vi "event_setup_start.vi"(7 "NewVal":bool, 8 "error in":errorcluster, 9 "reference cluster in":T1, 11 "Boolean in":refnum<vi>) -> (0 "error out":errorcluster)   [LabVIEW 2016]
uses:
  Type Definitions/reference_cluster.ctl
  Type Definitions/vars_settings.ctl
  Type Definitions/stim_type.ctl
  Type Definitions/backlight_type.ctl
  Type Definitions/vars_runtime.ctl
  Type Definitions/data.ctl
  Type Definitions/notifier_elements_GUI.ctl
  Type Definitions/notifier_elements_DAQ.ctl
  Type Definitions/notifier_elements_write.ctl
  Type Definitions/control_references.ctl
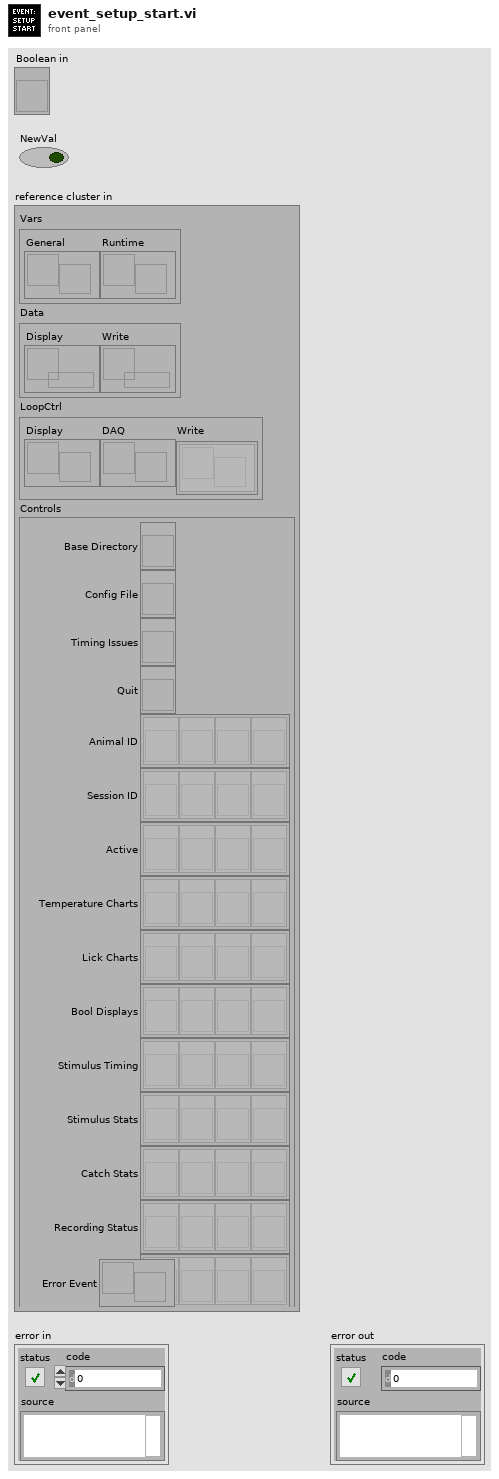
[diagram p1: front panel]
types:
  T1 = typedef "reference_cluster.ctl" = cluster{"Vars":cluster{"General":refnum<notifier>, "Runtime":refnum<notifier>}, "Data":cluster{"Display":refnum<queue>, "Write":refnum<queue>}, "LoopCtrl":cluster{"Display":refnum<notifier>, "DAQ":refnum<notifier>, "Write":refnum<notifier>[]}, "Controls":T2, "Error Event":refnum<user-event>}
  T2 = typedef "control_references.ctl" = cluster{"Base Directory":refnum<vi>, "Config File":refnum<vi>, "Timing Issues":refnum<vi>, "Quit":refnum<vi>, "Animal ID":refnum<vi>[], "Session ID":refnum<vi>[], "Active":refnum<vi>[], "Temperature Charts":refnum<vi>[], "Lick Charts":refnum<vi>[], "Bool Displays":refnum<vi>[], "Stimulus Timing":refnum<vi>[], "Stimulus Stats":refnum<vi>[], "Catch Stats":refnum<vi>[], "Recording Status":refnum<vi>[], "Pairing":refnum<vi>[]}
  T3 = enum8{"Enabled", "Disabled", "Disabled and Grayed Out"}
  T4 = typedef "notifier_elements_write.ctl" = enum16{"Initialize", "Pause", "Write Data", "Close Files", "Quit"}
  T5 = enum8{"Enabled", "Disabled", "Disabled and Grayed Out"}[]
  T6 = typedef "vars_settings.ctl" = cluster{"base directory":path, "data directory":path, "active":bool, "running":bool, "pairing":bool, "clean tubes":bool, "animal ID":u16, "session ID":u16, "base temp":dbl, "d wait min":u16, "d wait max":u16, "d timeout":u16, "d timeout catch":u16, "d penalty":u16, "d reward":u16, "n reward":u16, "idx stim":u16, "timeout win":u16, "lick win":i32[], "stim type":T7[], "stim dur":u16[], "stim amp":dbl[], "stim freq":u16[], "stim ramp":u16[], "stim catch":u8[], "pairing delay":i16[], "square dur":u16[], "square delay":i16[], "square freq":u8[], "square dc":u8[], "stim shape":dbl[][], "square shape":bool[][], "backlight type":T8, "backlight freq":u16, "dStimOne dur":u16[], "dStimOne delay":i16[], "dStimTwo dur":u16[], "dStimTwo delay":i16[]}
  T7 = typedef "stim_type.ctl" = enum16{"pulse", "vibration", "square", "sine"}
  T8 = typedef "backlight_type.ctl" = enum16{"none", "random", "regular"}
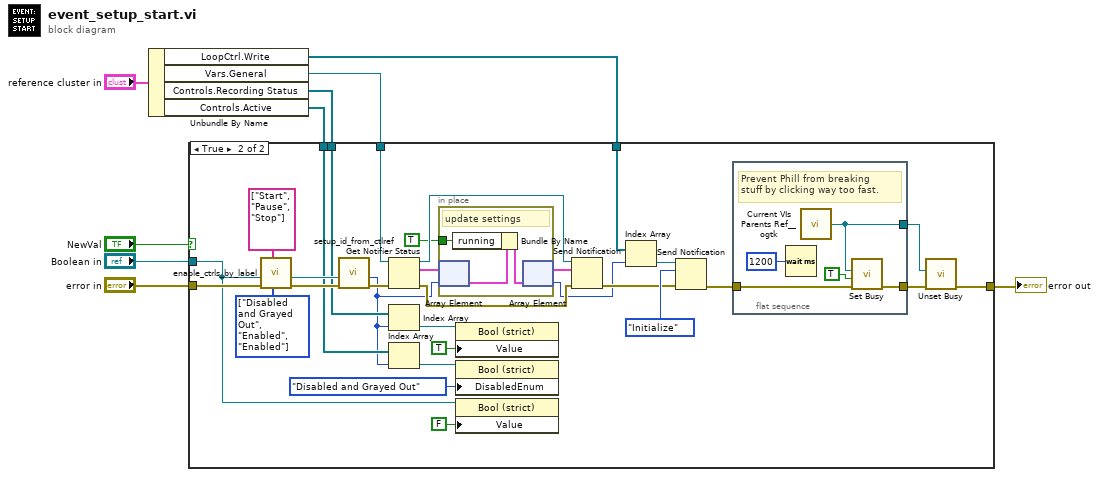
[diagram p0: block diagram]
diagram:
  n1 = Unbundle By Name("reference cluster in") -> ("LoopCtrl.Write"=w4:refnum<notifier>[], "Vars.General"=w7:refnum<notifier>, "Controls.Recording Status"=w8:refnum<vi>[], "Controls.Active"=w9:refnum<vi>[])
  n2 = case shown="True" "NewVal" {
    tunnel: [w10 w13] -> w1
    tunnel: "Boolean in" -> [_ w16]
    tunnel: "error in" -> [w10 w37]
    tunnel: w4 -> [_ w40]
    tunnel: w7 -> [_ w24]
    tunnel: w8 -> [_ w21]
    tunnel: w9 -> [_ w19]
    frame False {
    }
    frame True {
      w36 = T5 [enum."Disabled and Grayed Out", enum."Enabled", enum."Enabled"] items=["Enabled", "Disabled", "Disabled and Grayed Out"] ("State")
      n3 = call "enable_ctrls_by_label.vi"("States"=w36, "Names"=string[] ["Start", "Pause", "Stop"], "error in"=w37, "Refnum in"=w16) -> ("error out"=w27:errorcluster, "Refnum out"=w25:refnum<vi>)  [unwired: 6 in]
      n4 = call "setup_id_from_ctlref.vi"("error in"=w27, "Ctl Refnum"=w25) -> ("error out"=w26:errorcluster, "setup ID"=w18:u16)  [unwired: 6 in]
      n5 = Get Notifier Status(notifier=w24, error in (no error)=w26) -> (notifier out=w34:refnum<notifier>, current notification=w33:T6[], error out=w31:errorcluster)  [unwired: 2 out]
      n6 = Index Array(array=w21, index=w18) -> (element=w22:refnum<vi>)
      n7 = Index Array(array=w19, index=w18) -> (element=w20:refnum<vi>)
      n8 = in-place {
        in-place-border: TRUE ("NewVal") -> [w47]
        # "update settings"
        n9 = in-place-array #1(w33, w18) -> (w48:T6)
        n10 = Bundle By Name(cluster=w48, "running"=w47) -> (w46:T6)
        n11 = in-place-array #1(w46) -> (w32:T6[], w29:i32)
      }
      n12 = property class="Bool (strict)"(reference=w22, "Value"=TRUE) -> ()  [unwired: 1 in, 2 out]
      n13 = property class="Bool (strict)"(reference=w20, "DisabledEnum"=T3."Disabled and Grayed Out" ("Disabled")) -> ()  [unwired: 1 in, 2 out]
      n14 = property class="Bool (strict)"(reference=w16, "Value"=FALSE) -> ()  [unwired: 1 in, 2 out]
      n15 = Send Notification(notification=w32, notifier=w34, error in (no error)=w31) -> (error out=w30:errorcluster)  [unwired: 1 out]
      n16 = Index Array(array=w40, index=w29) -> (element=w39:refnum<notifier>)
      n17 = Send Notification(notification=notifier_elements_write."Initialize", notifier=w39, error in (no error)=w30) -> (error out=w14:errorcluster)  [unwired: 1 out]
      n18 = flat-sequence {
        tunnel: w14 -> [w44]
        tunnel: [w42] -> w12
        tunnel: [w41] -> w11
        frame #0 {
          # "Prevent Phill from breaking\nstuff by clicking way too fast."
          n19 = Wait (ms)(milliseconds to wait=u32 1200) -> ()  [unwired: 1 out]
          n20 = call <userlib>:"Current VIs Parents Ref__ogtk.vi"() -> ("Calling VI's Reference"=w41:refnum<vi>)  [unwired: 2 in]
          n21 = call <vilib>:"Set Busy.vi"("error in (no error)"=w44, "disable click? (T)"=TRUE, "VI reference (current VI)"=w41) -> ("error out"=w42:errorcluster)  [unwired: 7 in, 1 out]
        }
      }
      n22 = call <vilib>:"Unset Busy.vi"("error in (no error)"=w12, "VI reference (current VI)"=w11) -> ("error out"=w13:errorcluster)  [unwired: 9 in]
    }
  }
  "error out" <- w1
